vi "Init.vi"(6 "CW?":bool, 7 "RF Powers":dbl[](array[numeric]), 8 "error in (no error)":errorcluster, 9 "DC Pins":string[](array[string]), 10 "Measurement Name":string, 11 "SA Pin":string) -> (0 "error out":errorcluster, 3 "ModSweep Gain out":refnum<class "Power Sweep.lvclass">)   [LabVIEW 2018, in "SeqAuto Evaluations.lvlib" / "Power Sweep.lvclass"]
uses:
  Power Sweep.lvclass
  C:/Sequence Automation/Plugins/SeqAuto IEvaluation.lvlibp/SeqAuto IEvaluation.lvclass
  Power Sweep.lvclass/Power Sweep.ctl
  Plugins/SeqAuto IEvaluation.lvlibp/Write Measurement Name.vi
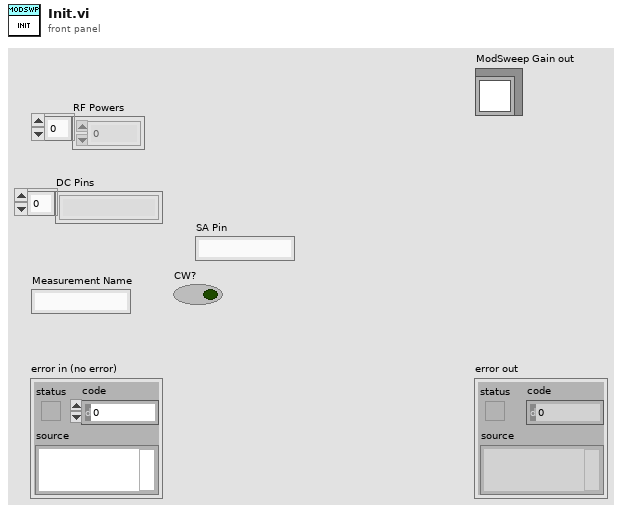
[diagram p1: front panel]
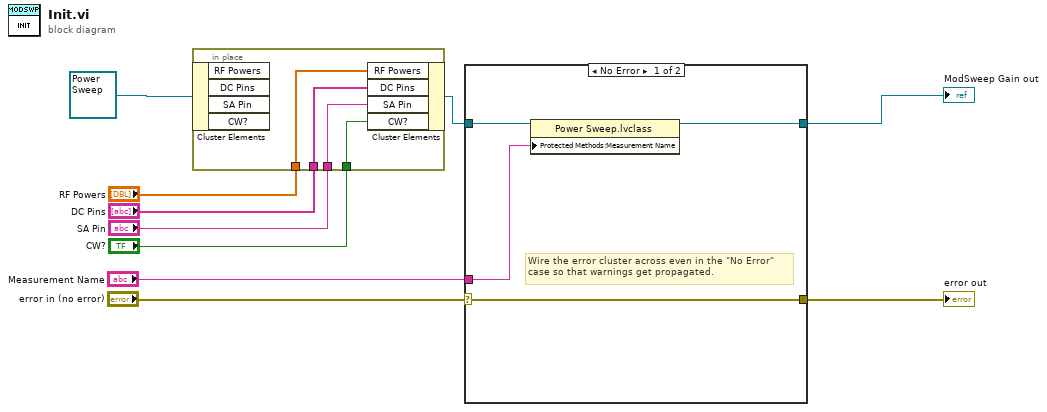
[diagram p0: block diagram]
diagram:
  n1 = in-place {
    in-place-border: "RF Powers" -> [w14]
    in-place-border: "DC Pins" -> [w13]
    in-place-border: "SA Pin" -> [w12]
    in-place-border: "CW?" -> [w11]
    n2 = in-place-cluster #1(refnum<class "Power Sweep.lvclass"> refnum ("ModSweep Gain in")) -> ()  [unwired: 4 out]
    n3 = in-place-cluster #1("RF Powers"=w14, "DC Pins"=w13, "SA Pin"=w12, "CW?"=w11) -> (w6:refnum<class "Power Sweep.lvclass">)
  }
  n4 = case shown="No Error" "error in (no error)" {
    selector: "error in (no error)" -> [w17 w20]
    tunnel: [w17 w20] -> w9
    tunnel: [w16 w19] -> w8
    tunnel: w6 -> [w18 w19]
    tunnel: "Measurement Name" -> [w15 _]
    frame No Error {
      # "Wire the error cluster across even in the \"No Error\"\ncase so that warnings get propagated."
      n5 = property class="Power Sweep.lvclass"(reference=w18, "Protected Methods:Measurement Name"=w15) -> (reference out=w16:refnum<class "Power Sweep.lvclass">)  [unwired: 1 in, 1 out]
    }
    frame Error {
    }
  }
  "error out" <- w9
  "ModSweep Gain out" <- w8
